vi "SAV.vi"(0 "System no.":i32=1 min=1 max=4 step=1, 2 "Axes to be saved":string[](array[string]), 3 "All axes?":bool, 4 "Axis identifier?":bool=TRUE, 5 "error in":errorcluster) -> (19 "error out":errorcluster)   [LabVIEW 2020]
doc: "Saves parameters of any of the specified axes which have been modified using SPA command.\n\nC-702: If All axes = TRUE, then Axis identifier must be TRUE. Save configuration of given axis. Saves the current stage configuration (stage-to-axis assignment with CST) and the corresponding motion parameter values (can be modified with SPA) from RAM to non-volatile memory and thus makes them the new power-on default.\nC-848: If All axes = TRUE, then Axis identifier must be TRUE\nC-880: If All axes = TRUE, then Axis identifier must be TRUE"
panel:
  # "Saves parameters of specified axes which have\nbeen modified using command SPA."
  # "If all axes: use"
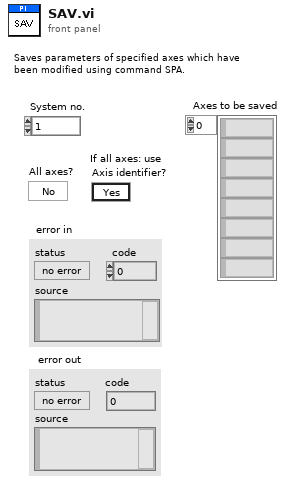
[diagram p1: front panel]
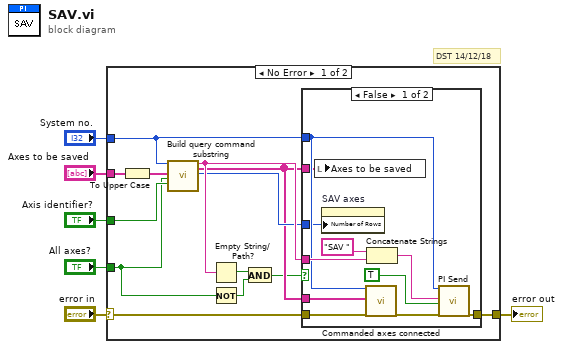
[diagram p0: block diagram]
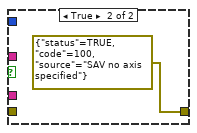
[diagram p2: hidden frame]
diagram:
  # "DST 14/12/18"
  n1 = case shown="No Error" "error in" {
    selector: "error in" -> [w9 w32]
    tunnel: "Axes to be saved" -> [w19 _]
    tunnel: "Axis identifier?" -> [w17 _]
    tunnel: "System no." -> [w15 _]
    tunnel: "All axes?" -> [w12 _]
    tunnel: [w10 w32] -> w2
    frame No Error {
      n2 = To Upper Case(1:w19) -> (0:w18:string[])
      n3 = call "Build query command substring.vi"("System no."=w15, "Axes to query in"=w18, "Query\nAll axes?"=w12, "For all axes: use\nAxis identifier?"=w17) -> ("Command substring"=w16:string, "Axes to query out"=w8:string[], "Number of rows"=w14:u32)  [unwired: 2 in, 11 out]
      n4 = Empty String/Path?(string/path=w16) -> (empty?=w13:bool)
      n5 = Not(x=w12) -> (.not. x?=w11:bool)
      n6 = And(x=w13, y=w11) -> (x .and. y?=w7:bool)
      n7 = case shown="False" w7 {
        tunnel: w16 -> [w27 _]
        tunnel: w15 -> [w26 _]
        tunnel: w14 -> [w24 _]
        tunnel: [w20 errorcluster {"status"=TRUE, "code"=100, "source"="SAV no axis specified"} ("error out")] -> w10
        tunnel: w9 -> [w23 _]
        tunnel: w8 -> [w22 _]
        tunnel: w8 -> [w21 _]
        frame False {
          n8 = local write "Axes to be saved"(w21) -> ()
          n9 = property on="SAV axes" class="Arr (strict)"("Number of Rows"=w24) -> ()  [unwired: 2 in, 2 out]
          n10 = call "Commanded axes connected.vi"("System no."=w26, "Commanded axes"=w22, "error in"=w23) -> ("error out"=w25:errorcluster)  [unwired: 1 in, 15 out]
          n11 = Concatenate Strings("SAV ", w27) -> (w28:string)
          n12 = call "PI Send.vi"("System no."=w26, "String to send"=w28, "Attach termination char.?"=TRUE ("Attach Linefeed?"), "error in"=w25) -> ("error out"=w20:errorcluster)  [unwired: 2 in, 13 out]
        }
        frame True {
        }
      }
    }
    frame Error {
    }
  }
  "error out" <- w2
